vi "String to 1D Array__ogtk.vi"(5 "ignore duplicate delimiters? (F=No)":bool, 7 "delimiter (Tab)":string="\t", 10 "string":string) -> (1 "Array of Strings":string[](array[string]))   [LabVIEW 2019]
doc: "Converts delimited string to a 1D array."
panel:
  # "[OpenG VI Tags] ***Do Not Remove***"
  # "String to 1D Array.vi\n\nConverts delimited string to a 1D array.\n\nPlease visit http://www.OpenG.org to learn about the\nOpen Source LabVIEW software movement.\n\nNOTICE -- YOU MUST LEAVE THIS NOTICE IN PLACE.  PER THE TERMS OF THE LICENSE BELOW, YOU MAY SUBLICENSE THIS SOFTWARE \nIN ANY WAY THAT DOES NOT CONFLICT WITH THIS LICENSE.\n\n### BSD License (http://www.opensource.org/licenses/bsd-license.php) Begin ###\n \nCopyright (c) 2002, Jim Kring <jim@jimkring.com>\nCopyright (c) 2005, MKS Instruments, Inc., author: Doug Femec<doug_femec@mksinst.com>, IM dafemec\n\nAll rights reserved.\n\nRedistribution and use in source and binary forms, with or without modification, are permitted provided that the following conditions are met:\n\n    * Redistributions of source code must retain the above copyright notice, this list of conditions and the following disclaimer.\n    * Redistributions in binary form must reproduce the above copyright notice, this list of conditions and the following disclaimer in the \n       documentation and/or other materials provided with the distribution.\n    * Neither the name of SciWare, James Kring, Inc., nor the names of its contributors may be used to endorse or promote products derived \n       from this software without specific prior written permission.\n\nTHIS SOFTWARE IS PROVIDED BY THE COPYRIGHT HOLDERS AND CONTRIBUTORS \"AS IS\" AND ANY EXPRESS OR IMPLIED WARRANTIES, \nINCLUDING, BUT NOT LIMITED TO, THE IMPLIED WARRANTIES OF MERCHANTABILITY AND FITNESS FOR A PARTICULAR PURPOSE ARE \nDISCLAIMED. IN NO EVENT SHALL THE COPYRIGHT OWNER OR CONTRIBUTORS BE LIABLE FOR ANY DIRECT, INDIRECT, INCIDENTAL,\n SPECIAL, EXEMPLARY, OR CONSEQUENTIAL DAMAGES (INCLUDING, BUT NOT LIMITED TO, PROCUREMENT OF SUBSTITUTE GOODS OR \nSERVICES; LOSS OF USE, DATA, OR PROFITS; OR BUSINESS INTERRUPTION) HOWEVER CAUSED AND ON ANY THEORY OF LIABILITY, \nWHETHER IN CONTRACT, STRICT LIABILITY, OR TORT (INCLUDING NEGLIGENCE OR OTHERWISE) ARISING IN ANY WAY OUT OF THE USE \nOF THIS SOFTWARE, EVEN IF ADVISED OF THE POSSIBILITY OF SUCH DAMAGE.\n\n### BSD License End ###"
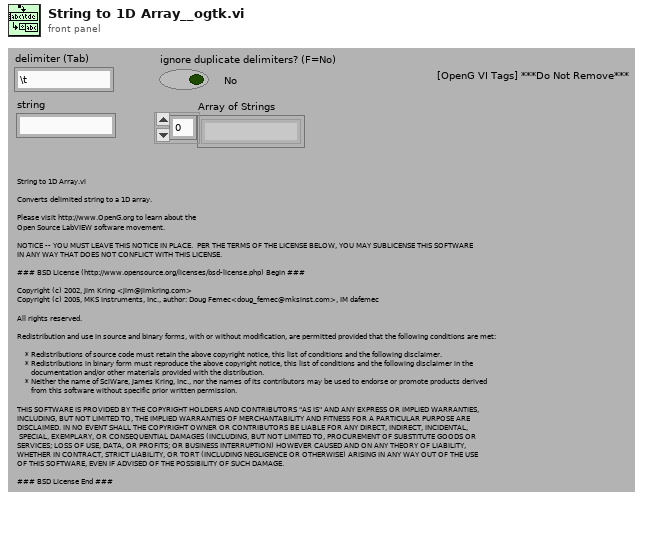
[diagram p1: front panel]
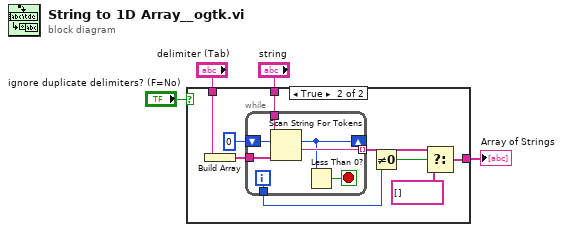
[diagram p0: block diagram]
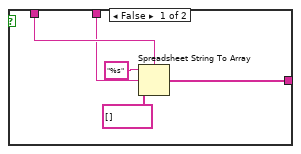
[diagram p2: hidden frame]
diagram:
  n1 = case shown="True" "ignore duplicate delimiters? (F=No)" {
    tunnel: [w7 w11] -> w1
    tunnel: "delimiter (Tab)" -> [w6 w12]
    tunnel: "string" -> [w5 w10]
    frame False {
      n2 = Spreadsheet String To Array(delimiter (Tab)=w6, format string="%s", spreadsheet string=w5, array type (2D Dbl)=string[] [] ("Array Constant")) -> (array=w7:string[])
    }
    frame True {
      n3 = Build Array(w12) -> (w17:string[])
      n4 = while {
        shift-right: [w23] -> _
        shift-left: 0 ("offset past token") -> [w25]
        tunnel: [w24] -> w16 mode=indexing
        tunnel: w10 -> [w21]
        tunnel: w17 -> [w20]
        tunnel: [w19] -> w15
        i -> [w19]
        stop <- w22 stop-if-true
        n5 = Scan String For Tokens(6:w20, 8:w25, 9:w21) -> (1:w24:string, 2:w23:i32)  [unwired: 3 in, 2 out]
        n6 = Less Than 0?(x=w23) -> (x < 0?=w22:bool)
      }
      n7 = Not Equal To 0?(x=w15) -> (x != 0?=w14:bool)
      n8 = Select(t=w16, s=w14, f=string[] []) -> (s? t:f=w11:string[])
    }
  }
  "Array of Strings" <- w1
